vi "Set Cell (DBL).vi"(6 "Column":i32, 7 "Value":dbl, 8 "error in (no error)":errorcluster, 9 "Row":i32, 10 "Sheet Reference":refnum<k24>) -> (0 "error out":errorcluster, 2 "Sheet Reference out":refnum<k24>)   [LabVIEW 2014]
uses:
  C:/Users/LENOVO/Desktop/CodeSpace GUI/LVExcel/Resources/net40/NPOI.dll
  Resources/net40/NPOI.dll
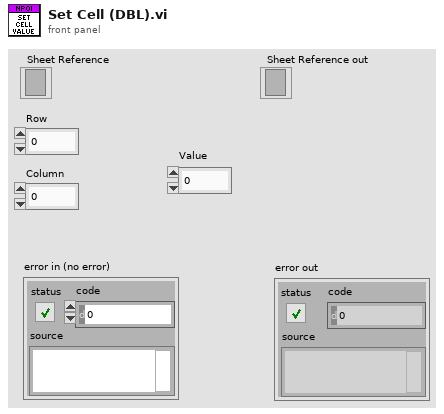
[diagram p1: front panel]
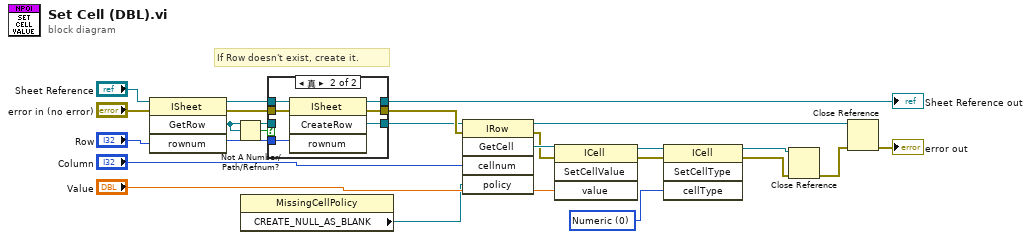
[diagram p0: block diagram]
diagram:
  w1 = 0 items=["Numeric"=0, "String"=1, "Formula"=2, "Blank"=3, "Boolean"=4, "Error"=5, "Unknown"=-1] ("cellType")
  # "If Row doesn't exist, create it."
  n1 = invoke class="ISheet" method="GetRow"(reference="Sheet Reference", error in="error in (no error)", "rownum"="Row") -> (reference out=w13:refnum<k24>, error out=w12:errorcluster, "GetRow"=w6:refnum<k24>)  [unwired: 1 in, 1 out]
  n2 = Not A Number/Path/Refnum?(number/path/refnum=w6) -> (NaN/Path/Refnum?=w7:bool)
  n3 = property class="MissingCellPolicy"() -> ("CREATE_NULL_AS_BLANK"=w14:refnum<k24>)  [unwired: 2 in, 2 out]
  n4 = case shown="真" w7 {
    tunnel: w13 -> [w26 w32]
    tunnel: w12 -> [w25 w31]
    tunnel: [w25 w30] -> w11
    tunnel: [w26 w29] -> w10
    tunnel: "Row" -> [_ w28]
    tunnel: [w24 w27] -> w8
    tunnel: w6 -> [w24 _]
    frame False {
    }
    frame True {
      n5 = invoke class="ISheet" method="CreateRow"(reference=w32, error in=w31, "rownum"=w28) -> (reference out=w29:refnum<k24>, error out=w30:errorcluster, "CreateRow"=w27:refnum<k24>)  [unwired: 1 in, 1 out]
    }
  }
  "Sheet Reference out" <- w10
  n6 = invoke class="IRow" method="GetCell"(reference=w8, error in=w11, "cellnum"="Column", "policy"=w14) -> (reference out=w21:refnum<k24>, error out=w18:errorcluster, "GetCell"=w19:refnum<k24>)  [unwired: 1 in, 2 out]
  n7 = invoke class="ICell" method="SetCellValue"(reference=w19, error in=w18, "value"="Value") -> (reference out=w5:refnum<k24>, error out=w4:errorcluster)  [unwired: 1 in, 2 out]
  n8 = invoke class="ICell" method="SetCellType"(reference=w5, error in=w4, "cellType"=w1) -> (reference out=w2:refnum<k24>, error out=w3:errorcluster)  [unwired: 1 in, 2 out]
  n9 = Close Reference(reference=w2, error in (no error)=w3) -> (error out=w17:errorcluster)
  n10 = Close Reference(reference=w21, error in (no error)=w17) -> (error out=→"error out":errorcluster)
